vi "Reload Data Type Information Collection.vi"(8 "error in (no error)":errorcluster, 11 "TwinCAT ADS in":refnum<class "TwinCAT ADS.lvclass">) -> (0 "error out":errorcluster, 3 "TwinCAT ADS out":refnum<class "TwinCAT ADS.lvclass">)   [LabVIEW 2018, in "TwinCAT ADS.lvclass"]
uses:
  TwinCAT ADS.lvclass
  TwinCAT ADS.lvclass/TwinCAT ADS.ctl
  TwinCAT.Ads
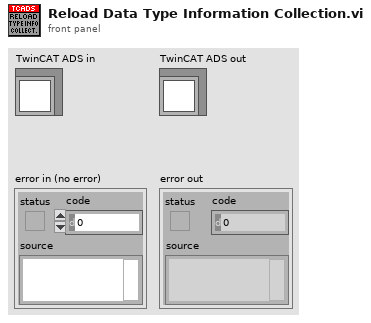
[diagram p1: front panel]
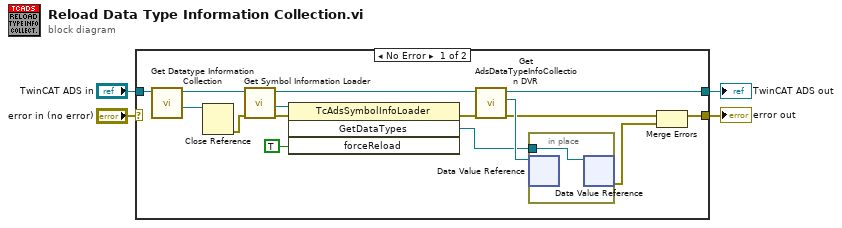
[diagram p0: block diagram]
diagram:
  n1 = case shown="No Error" "error in (no error)" {
    selector: "error in (no error)" -> [_ w22]
    tunnel: [w8 w22] -> w3
    tunnel: [w7 w21] -> w1
    tunnel: "TwinCAT ADS in" -> [w17 w21]
    frame No Error {
      n2 = call "Get Datatype Information Collection.vi"("TwinCAT ADS in"=w17) -> (".NET AdsDatatypeInfoCollection"=w16:refnum<k24>, "TwinCAT ADS out"=w6:refnum<class "TwinCAT ADS.lvclass">)  [unwired: 8 in, 1 out]
      n3 = Close Reference(reference=w16) -> (error out=w15:errorcluster)  [unwired: 1 in]
      n4 = call "Get Symbol Information Loader.vi"("error in (no error)"=w15, "TwinCAT ADS in"=w6) -> ("error out"=w19:errorcluster, ".NET AdsSymbolInfoLoader"=w5:refnum<k24>, "TwinCAT ADS out"=w13:refnum<class "TwinCAT ADS.lvclass">)  [unwired: 7 in]
      n5 = invoke class="TcAdsSymbolInfoLoader" method="GetDataTypes"(reference=w5, error in=w19, "forceReload"=TRUE) -> (error out=w14:errorcluster, "GetDataTypes"=w11:refnum<k24>)  [unwired: 1 in, 2 out]
      n6 = call "Get AdsDataTypeInfoCollection DVR.vi"("error in (no error)"=w14, "TwinCAT ADS in"=w13) -> ("error out"=w10:errorcluster, "AdsDatatypeInfoCollection DVR"=w12:refnum<data-value>, "TwinCAT ADS out"=w7:refnum<class "TwinCAT ADS.lvclass">)  [unwired: 7 in]
      n7 = in-place {
        in-place-border: w11 -> [w20]
        n8 = in-place-dvr #1(w12) -> ()  [unwired: 2 out]
        n9 = in-place-dvr #1(w20) -> (w9:errorcluster)  [unwired: 1 out]
      }
      n10 = Merge Errors(w10, w9) -> (w8:errorcluster)
    }
    frame Error {
    }
  }
  "error out" <- w3
  "TwinCAT ADS out" <- w1
